vi "wait for all modules to load.vi"(8 "error in (no error)":errorcluster) -> (0 "error out":errorcluster)   [LabVIEW 2012]
uses:
  GFG/GFGstringGet.vi
  GFG/GFG library.lvlib
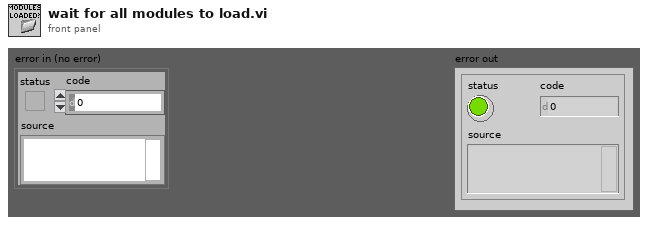
[diagram p1: front panel]
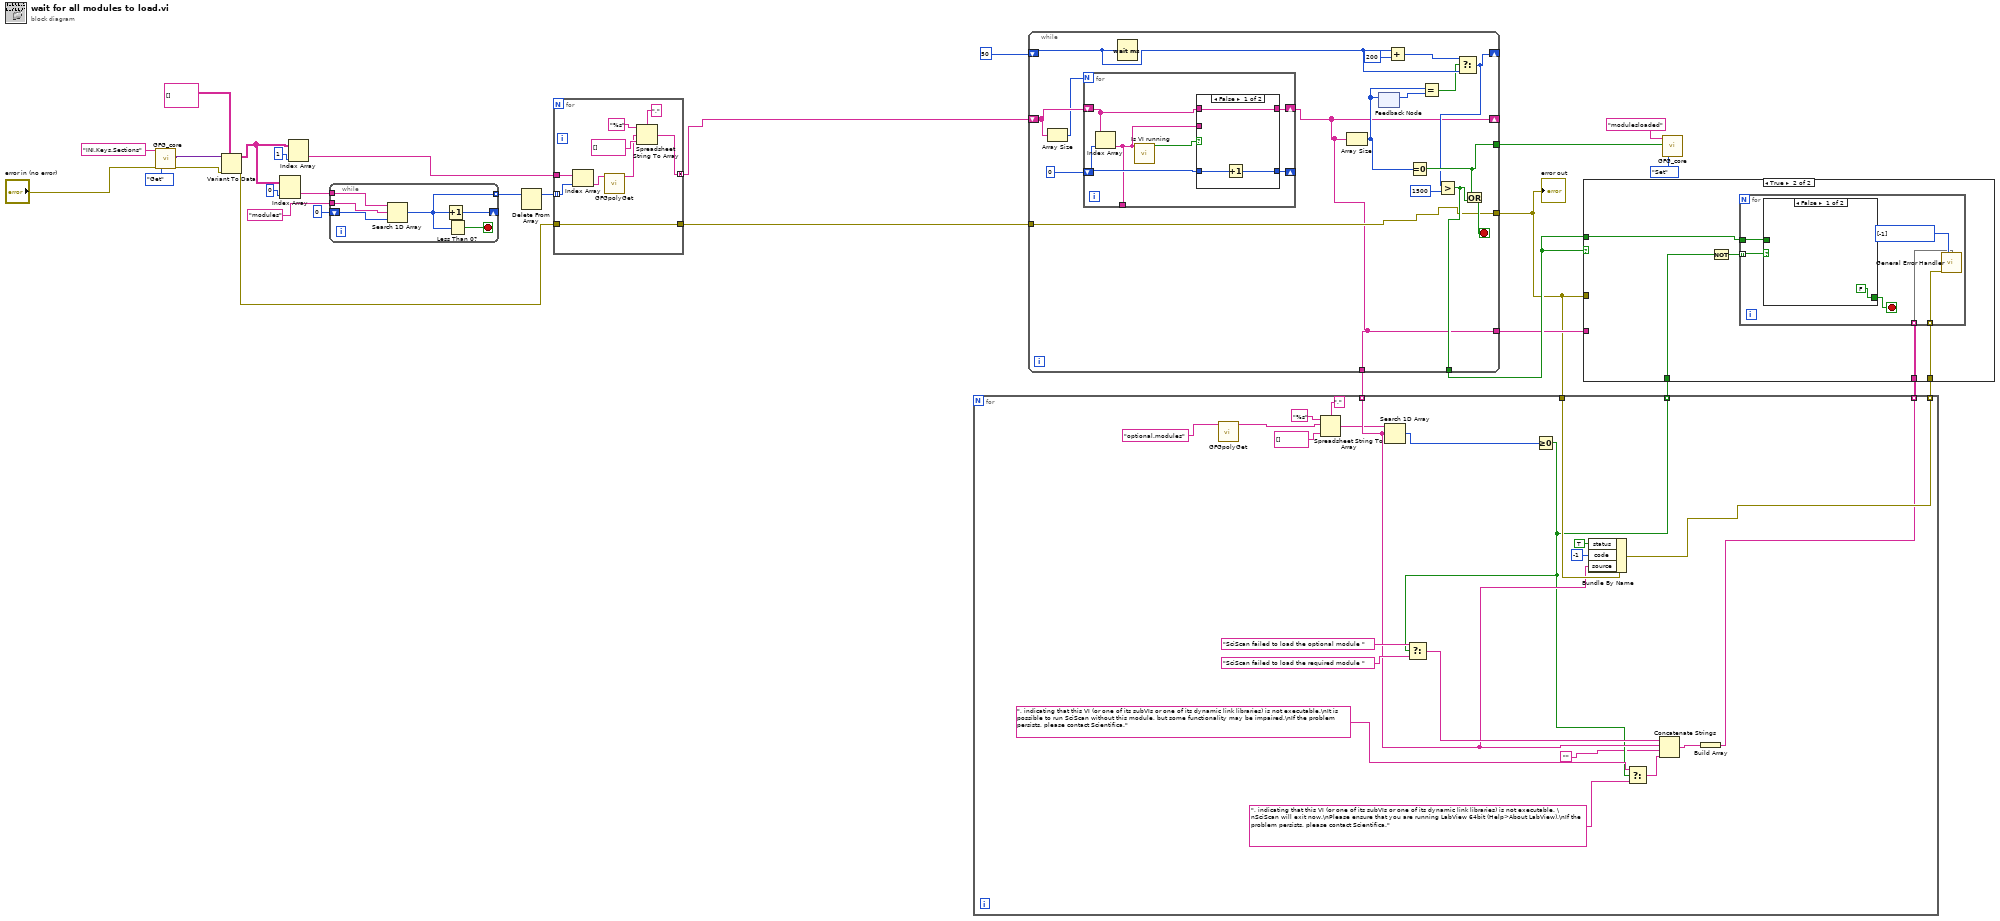
[diagram p0: block diagram]
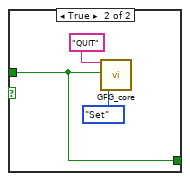
[diagram p3: hidden frame]
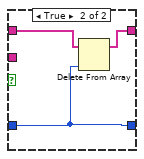
[diagram p4: hidden frame]
diagram:
  n1 = call "GFG_core.vi"("Variable Name in"="INI.Keys.Sections", "error in (no error)"="error in (no error)", "Action"=enum16{"Init", "Set", "Get"}."Get") -> ("Variant Out"=w27:variant, "error out"=w18:errorcluster)  [unwired: 10 in, 5 out]
  n2 = Variant To Data(error in=w18, type=string[][] [], Variant=w27) -> (data=w8:string[][], error out=w17:errorcluster)
  n3 = Index Array(array=w8, index (col)=0 ("index (row)")) -> (element=w6:string[])  [unwired: 1 in]
  n4 = Index Array(array=w8, index (col)=1 ("index (row)")) -> (element=w7:string[])  [unwired: 1 in]
  n5 = while {
    tunnel: w6 -> [w35]
    shift-right: [w32] -> _
    shift-left: 0 ("index of element") -> [w34]
    tunnel: [w31] -> w21 mode=indexing
    tunnel: "modules" ("element") -> [w30]
    stop <- w33 stop-if-true
    n6 = Search 1D Array(1D array=w35, element=w30, start index (0)=w34) -> (index of element=w31:i32)
    n7 = Increment(x=w31) -> (x+1=w32:i32)
    n8 = Less Than 0?(x=w31) -> (x < 0?=w33:bool)
  }
  n9 = Delete From Array(array=w21) -> (array with subset deleted=w20:i32[])  [unwired: 2 in, 1 out]
  n10 = for {
    tunnel: w7 -> [w44]
    tunnel: w20 -> [w43] mode=indexing
    tunnel: w17 -> [w36]
    tunnel: [w37] -> w16 mode=concatenating
    tunnel: [w36] -> w15
    n11 = Index Array(array=w44, index=w43) -> (element=w39:string)
    n12 = call-poly "GFGpolyGet.vi"("Variable Name in"=w39) -> ("String"=w38:string)  [unwired: 10 in]
    n13 = Spreadsheet String To Array(delimiter (Tab)=",", format string="%s" ("Variable Name in"), spreadsheet string=w38, array type (2D Dbl)=string[] [] ("Array")) -> (array=w37:string[])
  }
  n14 = while {
    shift-right: [w45] -> _
    shift-left: w16 -> [w60]
    tunnel: w15 -> [w46]
    tunnel: [w46] -> w5
    tunnel: [w57] -> w12
    shift-right: [w49] -> _
    shift-left: u32 50 ("milliseconds to wait") -> [w52]
    tunnel: [w47] -> w10
    tunnel: [w45] -> w9
    tunnel: [w45] -> w4
    stop <- w50 stop-if-true
    n15 = Array Size(array=w60) -> (size(s)=w59:i32)
    n16 = for {
      N: w59 -> [_]
      shift-right: [w65] -> w45
      shift-left: w60 -> [w64]
      shift-right: [w62] -> _
      shift-left: 0 -> [w63]
      tunnel: [w61] -> _
      n17 = Index Array(array=w64, index=w63) -> (element=w61:string)
      n18 = call "Is VI running.vi"("VI name"=w61) -> ("VI is running"=w66:bool)  [unwired: 9 in, 1 out]
      n19 = case shown="False" w66 {
        tunnel: w64 -> [w69 w72]
        tunnel: [w69 w70] -> w65
        tunnel: w61 -> [_ _]
        tunnel: w63 -> [w68 w71]
        tunnel: [w67 w71] -> w62
        frame False {
          n20 = Increment(x=w68) -> (x+1=w67:i32)
        }
        frame True {
          n21 = Delete From Array(array=w72, index=w71) -> (array with subset deleted=w70:string[])  [unwired: 1 in, 1 out]
        }
      }
    }
    n22 = Wait (ms)(milliseconds to wait=w52) -> ()  [unwired: 1 out]
    n23 = Array Size(array=w45) -> (size(s)=w56:i32)
    n24 = feedback-in #1(w56) -> ()
    n25 = feedback #1() -> (w55:i32)  [unwired: 1 in]
    n26 = Add(x=w52, y=u32 200) -> (x+y=w53:u32)
    n27 = Equal To 0?(x=w56) -> (x = 0?=w57:bool)
    n28 = Equal?(x=w56, y=w55) -> (x = y?=w51:bool)
    n29 = Select(t=w53, s=w51, f=w52) -> (s? t:f=w49:u32)
    n30 = Greater?(x=w49, y=u32 1500) -> (0:w47:bool)
    n31 = Or(x=w57, y=w47) -> (x .or. y?=w50:bool)
  }
  "error out" <- w5
  n32 = for {
    tunnel: w5 -> [w91]
    tunnel: w4 -> [w84] mode=indexing
    tunnel: [w83] -> w3 mode=indexing
    tunnel: [w74] -> w2 mode=indexing
    tunnel: [w73] -> w1 mode=indexing
    n33 = call-poly "GFGpolyGet.vi"("Variable Name in"="optional.modules" ("y")) -> ("String"=w77:string)  [unwired: 10 in]
    n34 = Spreadsheet String To Array(delimiter (Tab)=",", format string="%s" ("Variable Name in"), spreadsheet string=w77, array type (2D Dbl)=string[] [] ("Array")) -> (array=w76:string[])
    n35 = Search 1D Array(1D array=w76, element=w84) -> (index of element=w75:i32)  [unwired: 1 in]
    n36 = Greater Or Equal To 0?(x=w75) -> (x >= 0?=w83:bool)
    n37 = Select(t="SciScan failed to load the optional module " ("source"), s=w83, f="SciScan failed to load the required module " ("source")) -> (s? t:f=w86:string)
    n38 = Bundle By Name(cluster=w91, "status"=TRUE, "code"=-1, "source"=w84) -> (w74:errorcluster)
    n39 = Select(t=", indicating that this VI (or one of its subVIs or one of its dynamic link libraries) is not executable.\nIt is possible to run SciScan without this module, but some functionality may be impaired.\nIf the problem persists, please contact Scientifica." ("string"), s=w83, f=", indicating that this VI (or one of its subVIs or one of its dynamic link libraries) is not executable. \nSciScan will exit now.\nPlease ensure that you are running LabView 64bit (Help>About LabView).\nIf the problem persists, please contact Scientifica." ("string")) -> (s? t:f=w85:string)
    n40 = Concatenate Strings(w86, w84, "", w85) -> (w93:string)
    n41 = Build Array(w93) -> (w73:string[])
  }
  n42 = case shown="True" w10 {
    tunnel: w10 -> [_ w99]
    tunnel: w5 -> [_ _]
    tunnel: w9 -> [_ _]
    tunnel: w3 -> [_ w98]
    tunnel: w2 -> [_ w96]
    tunnel: w1 -> [_ w95]
    frame False {
    }
    frame True {
      n43 = Not(x=w98) -> (.not. x?=w97:bool[])
      n44 = for {
        tunnel: w99 -> [w105]
        tunnel: w97 -> [w104] mode=indexing
        tunnel: w96 -> [w101] mode=indexing
        tunnel: w95 -> [w100] mode=indexing
        stop <- w103 stop-if-true
        n45 = case shown="False" w104 {
          tunnel: w105 -> [_ w107]
          tunnel: [FALSE w107] -> w103
          frame False {
          }
          frame True {
            n46 = call "GFG_core.vi"("Variable Name in"="QUIT", "Variant in"=w107, "Action"=enum16{"Init", "Set", "Get"}."Set") -> ()  [unwired: 10 in, 7 out]
          }
        }
        n47 = call <vilib>:"General Error Handler.vi"("[user-defined codes]"=i32[] [-1], "[user-defined descriptions]"=w100, "error in (no error)"=w101) -> ()  [unwired: 8 in, 5 out]
      }
    }
  }
  n48 = call "GFG_core.vi"("Variable Name in"="modulesloaded", "Variant in"=w12, "Action"=enum16{"Init", "Set", "Get"}."Set") -> ()  [unwired: 10 in, 7 out]
